vi "Host_9.vi"() -> ()   [LabVIEW 2020]
uses:
  <vilib>/regexp/Match Regular Expression.xnode
panel:
  in  "stop":bool
  out "Dane":waveform(dbl)(graph)
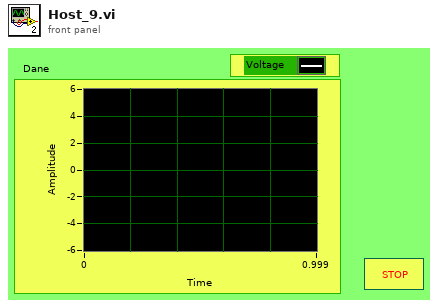
[diagram p1: front panel]
types:
  T1 = enum16{"open", "replace", "create", "open or create", "replace or create", "replace or create with confirmation"}
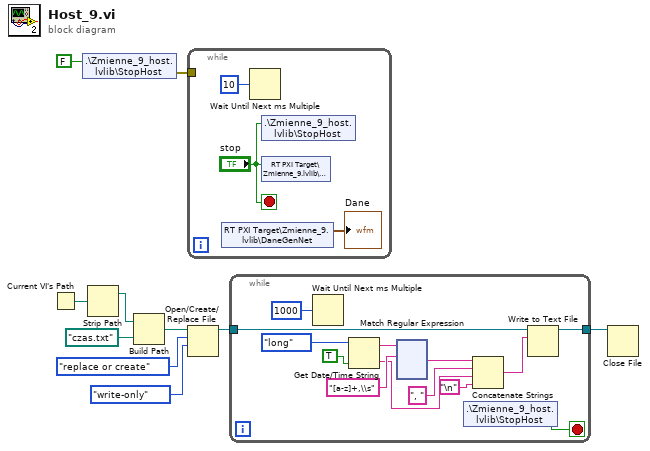
[diagram p0: block diagram]
diagram:
  n1 = Current VI's Path() -> (path=w5:path)
  n2 = shared-variable ".\\Zmienne_9_host.lvlib\\StopHost"(FALSE ("StopHost")) -> (error out=w1:errorcluster)  [unwired: 1 in]
  n3 = Strip Path(path=w5) -> (stripped path=w4:path)  [unwired: 1 out]
  n4 = Build Path(base path=w4, name or relative path=path "czas.txt") -> (appended path=w8:path)
  n5 = while {
    tunnel: w1 -> [_]
    stop <- "stop" stop-if-true
    n6 = shared-variable "RT PXI Target\\Zmienne_9.lvlib\\DaneGenNet"() -> (→"Dane":waveform(dbl))  [unwired: 1 in, 1 out]
    n7 = Wait Until Next ms Multiple(millisecond multiple=u32 10) -> ()  [unwired: 1 out]
    n8 = shared-variable ".\\Zmienne_9_host.lvlib\\StopHost"("stop") -> ()  [unwired: 1 in, 1 out]
    n9 = shared-variable "RT PXI Target\\Zmienne_9.lvlib\\Stop"("stop") -> ()  [unwired: 1 in, 1 out]
  }
  n10 = Open/Create/Replace File(file path (use dialog)=w8, operation (0:open)=T1."replace or create", access (0:read/write)=enum16{"read/write", "read-only", "write-only"}."write-only") -> (refnum out=w7:refnum<file>)  [unwired: 3 in, 2 out]
  n11 = while {
    tunnel: w7 -> [w22]
    tunnel: [w26] -> w6
    stop <- w18 stop-if-true
    n12 = Wait Until Next ms Multiple(millisecond multiple=u32 1000) -> ()  [unwired: 1 out]
    n13 = Get Date/Time String(date format (0)=enum16{"short", "long", "abbreviated"}."long", want seconds? (F)=TRUE) -> (date string=w20:string, time string=w15:string)  [unwired: 1 in]
    n14 = xnode "Match Regular Expression"("input string"=w20, "regular expression"="[a-z]+,\\s") -> ("after match"=w19:string)  [unwired: 4 in, 4 out]
    n15 = shared-variable ".\\Zmienne_9_host.lvlib\\StopHost"() -> (w18:bool)  [unwired: 1 in, 1 out]
    n16 = Concatenate Strings(w19, ", " ("string"), w15, "\n") -> (w17:string)
    n17 = Write to Text File(file (use dialog)=w22, text=w17) -> (refnum out=w26:refnum<file>)  [unwired: 2 in, 2 out]
  }
  n18 = Close File(refnum=w6) -> ()  [unwired: 1 in, 2 out]
